vi "CoilSim.vi"(8 "z(m)":dbl format="%#_13g", 9 "x(m)":dbl, 10 "zp(m)":dbl, 11 "I(A)":dbl) -> (2 "Bz(G)":dbl, 3 "Br(G)":dbl)   [LabVIEW 2012]
uses:
  <vilib>/gmath/SpecialFunctions.llb/Complete Elliptic Integral E.vi
  <vilib>/gmath/SpecialFunctions.llb/Complete Elliptic Integral K.vi
  <vilib>/gmath/NI_Gmath.lvlib
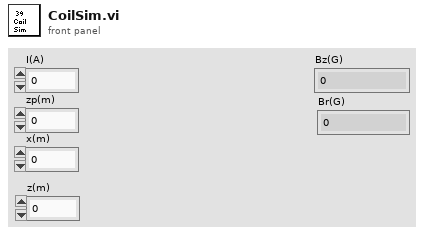
[diagram p1: front panel]
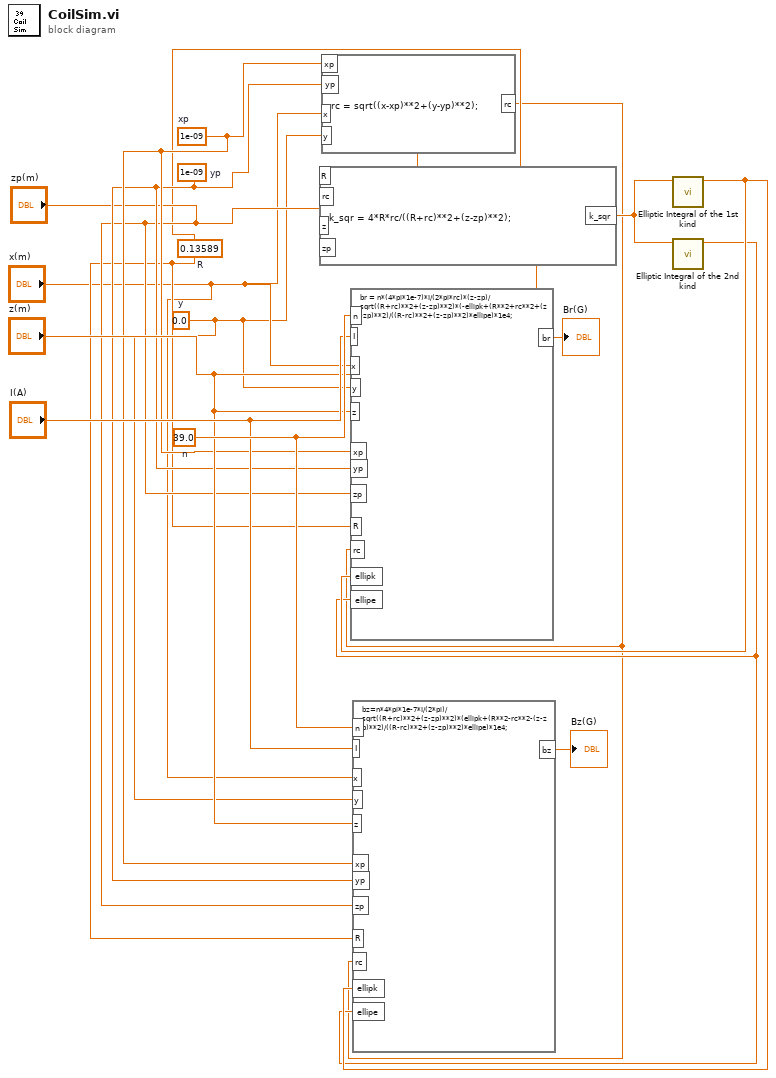
[diagram p0: block diagram]
diagram:
  w14 = 39.0  # n
  w8 = 0.13589  # R
  w3 = 0.0  # y
  w11 = 1e-09  # xp
  w10 = 1e-09  # yp
  n1 = formula code="rc = sqrt((x-xp)**2+(y-yp)**2);"("x"="x(m)", "y"=w3, "xp"=w11, "yp"=w10) -> ("rc"=w4:dbl)
  n2 = formula code="k_sqr = 4*R*rc/((R+rc)**2+(z-zp)**2);"("z"="z(m)", "zp"="zp(m)", "R"=w8, "rc"=w4) -> ("k_sqr"=w15:dbl)
  n3 = call-poly <vilib>:"Elliptic Integral of the 1st kind.vi"("k"=w15) -> ("K(k)"=w7:dbl)  [unwired: 10 in]
  n4 = call-poly <vilib>:"Elliptic Integral of the 2nd kind.vi"("k"=w15) -> ("E(k)"=w6:dbl)  [unwired: 10 in]
  n5 = formula code="br = n*(4*pi*1e-7)*I/(2*pi*rc)*(z-zp)/sqrt((R+rc)**2+(z-zp)**2)*(-ellipk+(R**2+rc**2+(z-zp)**2)/((R-rc)**2+(z-zp)**2)*ellipe)*1e4;"("x"="x(m)", "y"=w3, "n"=w14, "I"="I(A)", "z"="z(m)", "xp"=w11, "yp"=w10, "zp"="zp(m)", "R"=w8, "rc"=w4, "ellipk"=w7, "ellipe"=w6) -> ("br"=→"Br(G)":dbl)
  n6 = formula code="bz=n*4*pi*1e-7*I/(2*pi)/sqrt((R+rc)**2+(z-zp)**2)*(ellipk+(R**2-rc**2-(z-zp)**2)/((R-rc)**2+(z-zp)**2)*ellipe)*1e4;"("x"="x(m)", "y"=w3, "n"=w14, "I"="I(A)", "z"="z(m)", "xp"=w11, "yp"=w10, "zp"="zp(m)", "R"=w8, "rc"=w4, "ellipk"=w7, "ellipe"=w6) -> ("bz"=→"Bz(G)":dbl)
